vi "Calibration.vi"(4 "flush duration [s]":dbl, 6 "Exposure":sgl=50.0 format="%#_g ms", 7 "Desired Refresh Ratio":dbl=25.0 format="%#_g %", 8 "LINX Resource":T2={"IO"=enum."Remote", "Interface"=enum."TCP", "LINX Device Config"={"Interface"=enum."Serial", "COM Port"="COM13", "TCP Configuration"={"IP Address"="", "Port"=0}, "Device Family"=1, "Device ID"=1, "Device Name"="myRIO-1900", "TCP Ref"=refnum, "Channels"={"DI"=[0, 1, 2, 3, 4, 5, 6, 7, 8, 9, 10, 11, 12, 13, 14, 15, 16, 17, 18, 19, 20, 21, 22, 23, 24, 25, 26, 27, 28, 29, 30, 31, 32, 33, 34, 35, 36, 37, 38, 39, 40, 41, 42, 43, 44, 45, 46], "DO"=[0, 1, 2, 3, 4, 5, 6, 7, 8, 9, 10, 11, 12, 13, 14, 15, 16, 17, 18, 19, 20, 21, 22, 23, 24, 25, 26, 27, 28, 29, 30, 31, 32, 33, 34, 35, 36, 37, 38, 39, 40, 41, 42, 43, 44, 45, 46], "AI"=[0, 1, 2, 3, 4, 5, 6, 7, 8, 9, 10, 11], "AO"=[], "PWM"=[3, 5, 6, 9, 10], "QE"=[], "UART"=[0, 1], "I2C 2"=[0], "SPI"=[0], "CAN"=[], "Servo"=[], "AI Ref (V)"=0.0, "AI Resolution (Bits)"=0, "AO Ref (V)"=0.0, "AO Resolution (Bits)"=0}}}, 9 "SOLA ID":u32, 10 "TANGO ID":i32, 11 "IX 81 Port":refnum<visa-resource-name>="IX2-UCB") -> (0 "error IO":errorcluster, 2 "CalibFile":path, 3 "Number of pump steps\n for the desired refresh ratio":dbl)   [LabVIEW 2018]
doc: "This template is for the Queued Message Handler design pattern.\n\nThe Event Handling Loop generates messages based on user interface actions.\n\nThe Message Handling Loop processes messages generated by the Event Handling Loop, or by other messages. The messages are string values, so new messages can be added easily to the Message Cases case structure in the Message Handling Loop. Each message cluster can also provide an optional value for Message Data, which is a variant that can be converted to whatever message-specific data is required."
uses:
  <vilib>/MakerHub/LINX/Private/Type Defs/LINX Ref.ctl
  <vilib>/MakerHub/LINX/Private/Type Defs/Platform.ctl
  <vilib>/MakerHub/LINX/Private/Type Defs/Interface.ctl
  <vilib>/MakerHub/LINX/Private/Device/Type Defs/LINX Device Config.ctl
  <vilib>/MakerHub/LINX/Private/Device/Type Defs/TCP Config.ctl
  <vilib>/MakerHub/LINX/Private/Device/Type Defs/Channels.ctl
  C:/Users/johan/Downloads/LabVIEW software/LabVIEW software/IX-81 Software/lib/tiff/LVTiffWriter/BitMiracle.LibTiff.NET.dll
  lib/tiff/LVTiffWriter/BitMiracle.LibTiff.NET.dll
  <vilib>/MakerHub/LINX/Public/Peripherals/Digital/Digital Write N Chans.vi
  <vilib>/MakerHub/LINX/Private/Local IO/LinxDigitalWrite.vi
  <vilib>/MakerHub/LINX/Public/Utilities/Check Channel.vi
  <vilib>/MakerHub/LINX/Private/Utilties/Generate Error.vi
  lib/SOLA/LabVIEW 2015 Library (32bit)/LumencorDLL32/LumencorDLL32.lvlib
  lib/Olympus IX BX Series/Olympus IX BX Series.lvlib
  <vilib>/MakerHub/LINX/LMH-LINX.lvlib
  lib/ANDOR/Andor SDK/AndorSDK.lvlib
  <vilib>/vision/NI_Vision_Development_Module.lvlib
  lib/tiff/LVTiffWriter/LVTiffWriter.lvlib
  <vilib>/MakerHub/LINX/Private/Device/Device.lvlib
panel:
  out "function return":u32
  out "color":string
  in  "Messages":string
  out "TiffHandle":refnum<k24>
  in  "Image Name":string="TestIMG"
  out "Acq. Error Array":cluster{i32, string}[](array[cluster])
  in  "Single Image":bool
  out "Image":T1(plugin-control)
  in  "Colormap":u16(ring) items=["Grey", "Hot"]
  in  "Format":u16(ring)=6
  in  "Path":path
  in  "Save Image":bool
  in  "Exposure 2":sgl=50.0 format="%#_g ms"
  in  "Filter":u16(ring) items=["UV ", "CFP", "GFP", "YFP", "RFP", "BF (empty)"]
  out "exposure out":sgl
  out "accumulate out":sgl
  out "kinetic out":sgl
  out "Camera Temperature":sgl format="%.2f °C"
  in  "Calibrate at Startup":bool
  out "Y Limits":dbl[](array[numeric]) caption="Y Limits [µm]" format="%#_12f"
  out "X Limits":dbl[](array[numeric]) caption="X Limits [µm]" format="%#_10f"
  out "Lower Limit":dbl
  out "Upper Limit":dbl
  in  "Focus [um]":dbl format="%.3f"
  in  "Intensity [%]":dbl(slide) scale=0.0..100.0 scale format="%.1f"
  in  "Light Source":u16(ring) items=["BF - Lamp", "SOLA"]
  in  "Prism Position (1: Bi)":enum16{"Bi", "Side"}(ring)=enum."Side"
  in  "Objective":enum16{"x 4", "x 10", "x 20", "x 40", "x 100"}(ring)=enum."x 10"
  in  "Lamp Type (0: Transmitted)":enum16{"Transmitted", "Reflected"}(ring)
  in  "Enable Lamp":bool
  in  "Shutter":bool
  in  "Microscope Settings":i32(listbox)
  out "Slide":u8(slide) scale=0.0..100.0
  in  "Valve Actuation":i32(listbox)
  in  "Configuration File Path":path
  in  "stop":bool
  out "error out":errorcluster
  in  "Position List":i32[](listbox)
  out "Tango Success":bool
  in  "TANGO COM Port":refnum<visa-resource-name>="COM4"
  in  "SOLA COM Port":refnum<visa-resource-name>="COM5"
  in  "Valve Port (Arduino)":refnum<visa-resource-name>="COM7"
  # "Initialization"
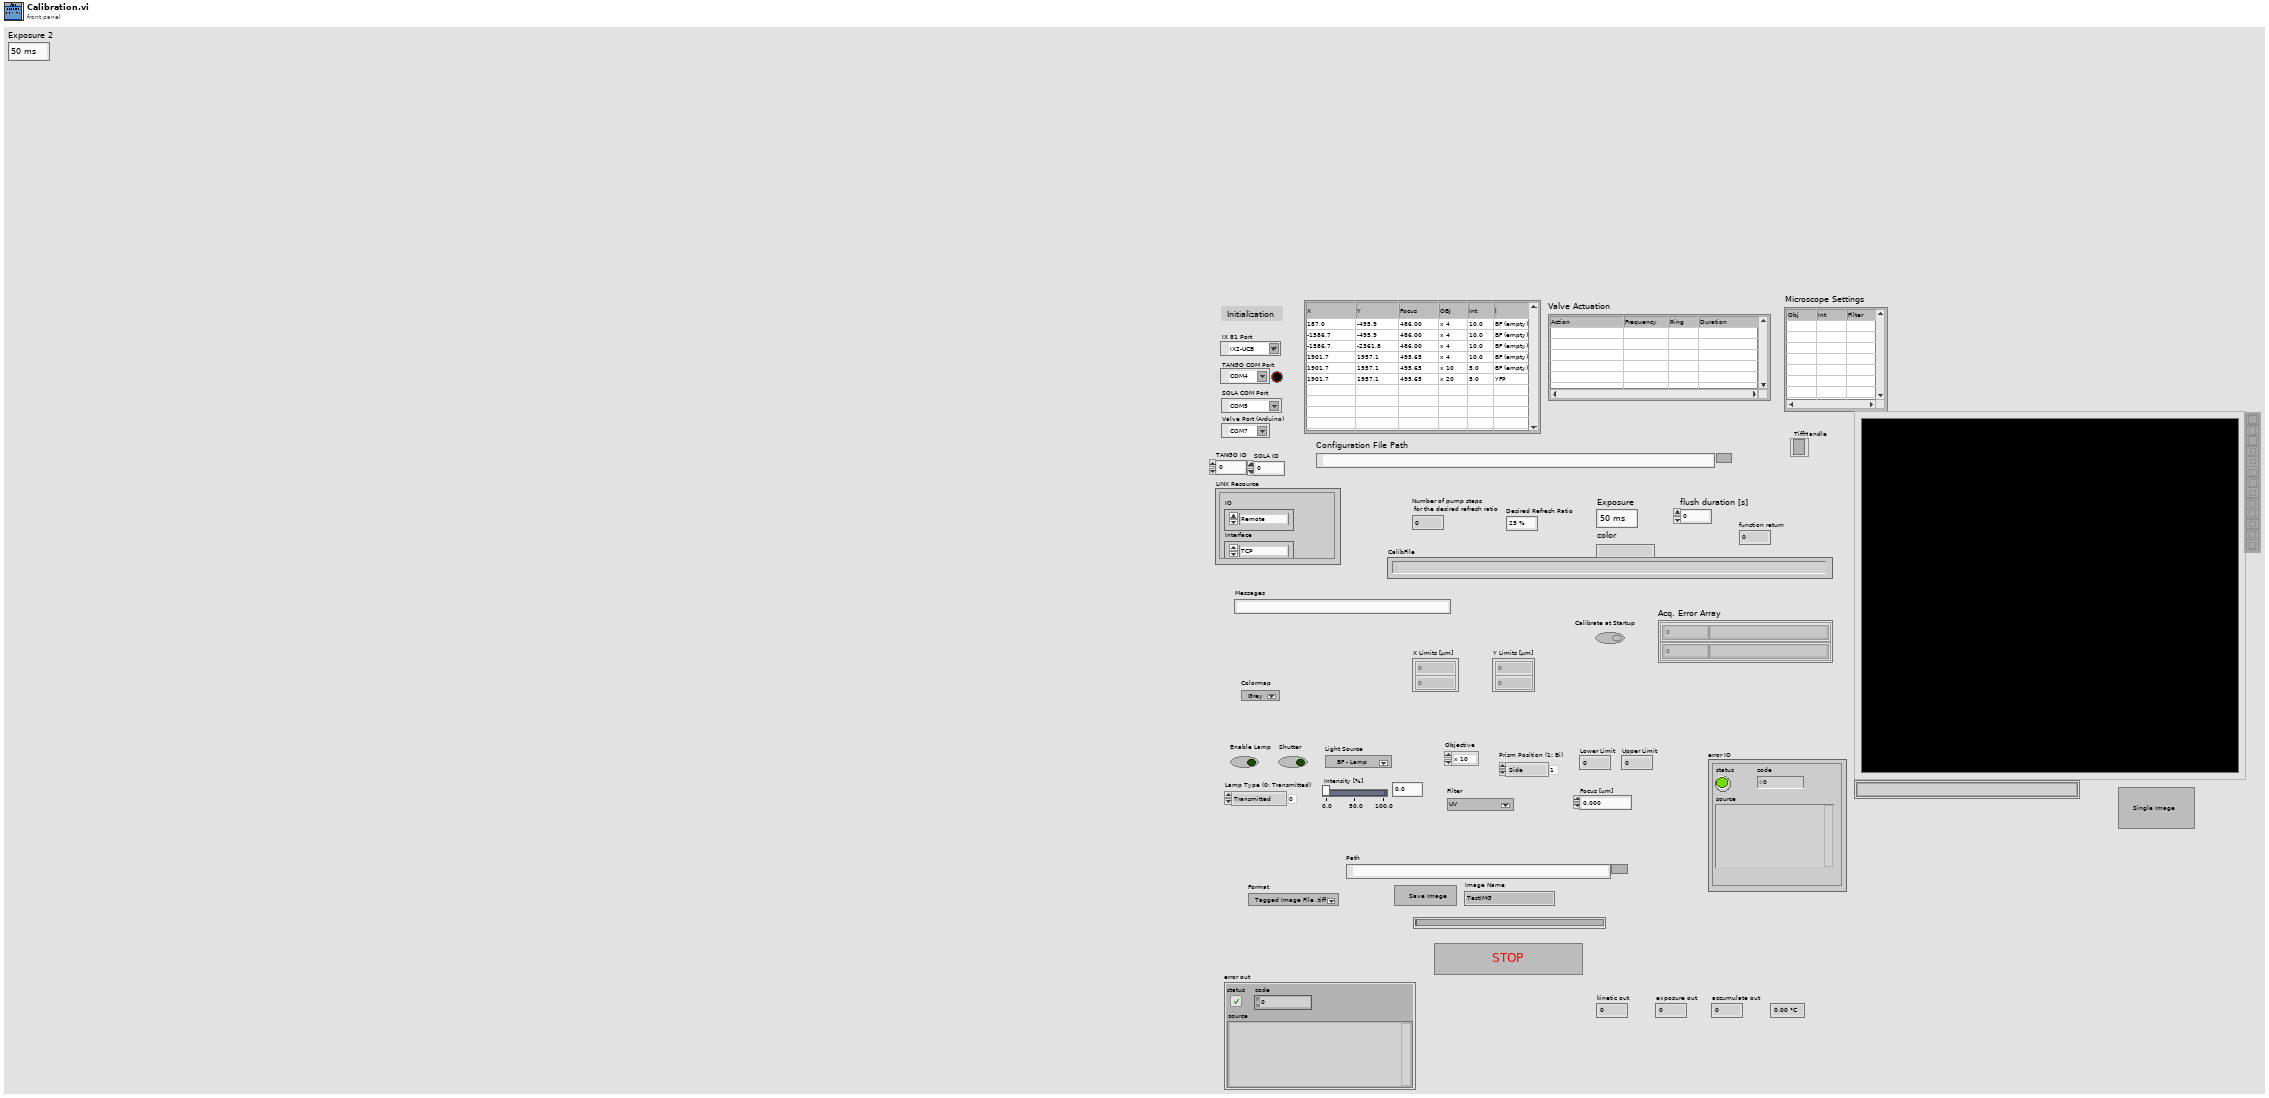
[diagram p1: front panel]
types:
  T1 = typedef "IMAQ Image.ctl" = refnum<image>
  T2 = typedef "LMH-LINX.lvlib/LINX Ref.ctl" = cluster{"IO":T3, "Interface":T4, "LINX Device Config":T5}
  T3 = typedef "LMH-LINX.lvlib/Platform.ctl" = enum16{"Remote", "Local"}
  T4 = typedef "LMH-LINX.lvlib/Interface.ctl" = enum16{"Serial", "TCP"}
  T5 = typedef "LMH-LINX.lvlib/Device.lvlib/LINX Device Config.ctl" = cluster{"Interface":T4, "COM Port":refnum<visa-resource-name>, "TCP Configuration":T6, "Device Family":u8, "Device ID":u8, "Device Name":string, "TCP Ref":refnum<k5>, "Channels":T7}
  T6 = typedef "LMH-LINX.lvlib/Device.lvlib/TCP Config.ctl" = cluster{"IP Address":string, "Port":u16}
  T7 = typedef "LMH-LINX.lvlib/Channels.ctl" = cluster{"DI":u8[], "DO":u8[], "AI":u8[], "AO":u8[], "PWM":u8[], "QE":u8[], "UART":u8[], "I2C 2":u8[], "SPI":u8[], "CAN":u8[], "Servo":u8[], "AI Ref (V)":dbl, "AI Resolution (Bits)":u8, "AO Ref (V)":dbl, "AO Resolution (Bits)":u8}
  T8 = enum16{"open", "replace", "create", "open or create", "replace or create", "replace or create with confirmation"}
  T9 = typedef "Image Type" = u32
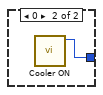
[diagram p2: hidden frame]
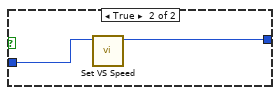
[diagram p3: hidden frame]
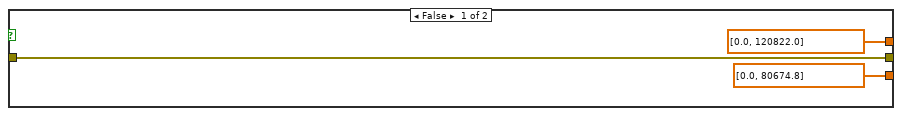
[diagram p4: hidden frame]
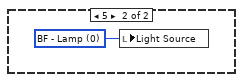
[diagram p5: hidden frame]
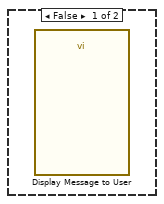
[diagram p7: hidden frame]
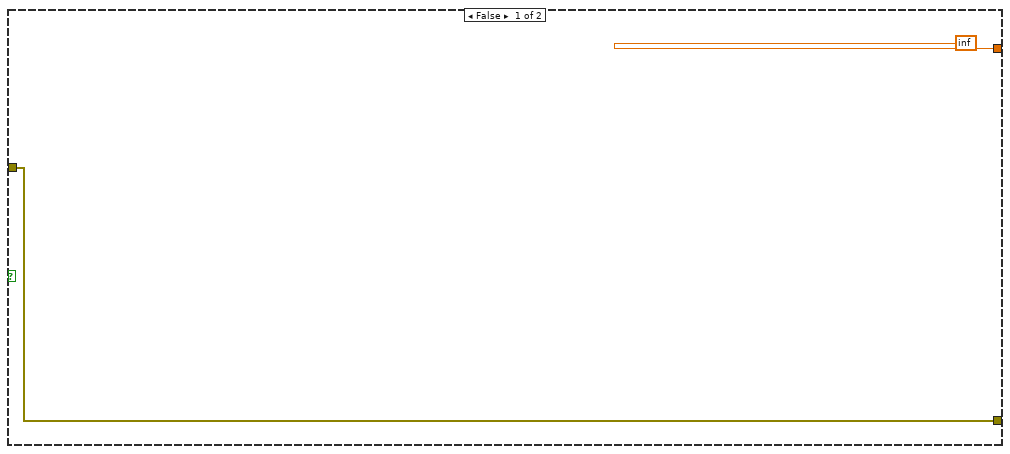
[diagram p11: hidden frame]
diagram:
  n1 = flat-sequence {
    tunnel: [errorcluster {"status"=FALSE, "code"=0, "source"=""} ("error IO")] -> w2
    tunnel: w2 -> [w5]
    tunnel: [w4] -> w1
    tunnel: w1 -> [_]
    frame #0 {
    }
    frame #1 {
      w70 = 0  # openingtime
      w68 = 0  # Auto Mode
      w67 = 1  # TTL High to open
      w69 = 0  # closingtime
      w66 = 0  # Internal Trigger
      w64 = 1  # Single Scan
      w65 = 4  # Image Read
      n2 = local read "IX 81 Port"() -> (w152:refnum<visa-resource-name>)
      n3 = call "Set Temperature.vi"("temperature"=-60) -> ()  [unwired: 10 in, 1 out]
      n4 = local write "Upper Limit"(3000000.0 ("default (0 I32)")) -> ()
      n5 = call "Set Active Objective.vi"("error in (no error)"=w5, "Objective Number (1)"=1, "Device Number (1)"=1, "VISA Resource Name"=w152) -> ("error out"=w103:errorcluster, "VISA Resource Name Out"=w104:refnum<visa-resource-name>)  [unwired: 6 in]
      n6 = local write "Lower Limit"(10.0 ("Upper Limit")) -> ()
      n7 = call "OlympusQuery.vi"("error in (no error)"=w103, "String"="SW OFF", "VISA Resource Name In"=w104) -> ("error out"=w107:errorcluster, "VISA Resource Name Out"=w108:refnum<visa-resource-name>)  [unwired: 6 in, 1 out]
      n8 = call "Is Cooler On.vi"() -> ("function return"=w53:u32, "iCoolerStatus out"=w54:i32)  [unwired: 10 in]
      n9 = call "OlympusQuery.vi"("error in (no error)"=w107, "String"="LMPSW OFF", "VISA Resource Name In"=w108) -> ("error out"=w102:errorcluster, "VISA Resource Name Out"=w149:refnum<visa-resource-name>)  [unwired: 6 in, 1 out]
      n10 = case shown="1, Default" w54 {
        tunnel: [u32 20002 ("function return") w161] -> w52
        frame 1, Default {
        }
        frame 0 {
          n11 = call "Cooler ON.vi"() -> ("function return"=w161:u32)  [unwired: 11 in]
        }
      }
      n12 = call "Get VS Speed.vi"() -> ("speed out"=w73:sgl, "function return"=w40:u32)  [unwired: 10 in]
      n13 = call "Get Fastest Recommended VS Speed.vi"() -> ("function return"=w39:u32, "speed out"=w72:sgl, "index out"=w75:i32)  [unwired: 9 in]
      n14 = Greater Or Equal?(x=w72, y=w73) -> (x >= y?=w74:bool)
      n15 = call "OlympusQuery.vi"("error in (no error)"=w102, "String"="LMP?", "VISA Resource Name In"=w149) -> ("error out"=w100:errorcluster, "Result"=w110:string, "VISA Resource Name Out"=w148:refnum<visa-resource-name>)  [unwired: 6 in]
      n16 = call "AndorCreaterErrorCluster.vi"() -> ("Array"=w38:cluster{i32, string}[])  [unwired: 11 in]
      n17 = case shown="False" w74 {
        tunnel: w75 -> [_ w164]
        tunnel: [u32 20002 ("function return") w163] -> w41
        frame False {
        }
        frame True {
          n18 = call "Set VS Speed.vi"("index"=w164) -> ("function return"=w163:u32)  [unwired: 10 in]
        }
      }
      n19 = call "AndorReturn2Error.vi"("Error List"=w38, "Camera return"=w53) -> ("error out"=w36:errorcluster, "Error List out"=w37:cluster{i32, string}[])  [unwired: 8 in]
      n20 = Decimal String To Number(string=w110, default (0L)=0.0 ("default (0 I32)")) -> (number=w112:dbl)  [unwired: 1 in, 1 out]
      n21 = call "AndorReturn2Error.vi"("error in (no error)"=w36, "Error List"=w37, "Camera return"=w52) -> ("error out"=w35:errorcluster, "Error List out"=w9:cluster{i32, string}[])  [unwired: 7 in]
      n22 = call "OlympusQuery.vi"("error in (no error)"=w100, "String"="SHUT1?", "VISA Resource Name In"=w148) -> ("error out"=w98:errorcluster, "Result"=w131:string, "VISA Resource Name Out"=w146:refnum<visa-resource-name>)  [unwired: 6 in]
      n23 = Divide(x=w112, y=1.2 ("x")) -> (x/y=w101:dbl)
      n24 = local write "Intensity [%]"(w101) -> ()
      n25 = call "AndorReturn2Error.vi"("error in (no error)"=w35, "Error List"=w9, "Camera return"=w39) -> ("error out"=w34:errorcluster, "Error List out"=w10:cluster{i32, string}[])  [unwired: 7 in]
      n26 = Equal?(x=w131, y="OUT") -> (x = y?=w99:bool)
      n27 = local write "Shutter"(w99) -> ()
      n28 = call "AndorReturn2Error.vi"("error in (no error)"=w34, "Error List"=w10, "Camera return"=w40) -> ("error out"=w33:errorcluster, "Error List out"=w11:cluster{i32, string}[])  [unwired: 7 in]
      n29 = call "OlympusQuery.vi"("error in (no error)"=w98, "String"="LMPSEL?", "VISA Resource Name In"=w146) -> ("error out"=w95:errorcluster, "Result"=w129:string, "VISA Resource Name Out"=w96:refnum<visa-resource-name>)  [unwired: 6 in]
      n30 = call "Get Temperature F.vi"() -> ("function return"=w42:u32, "temperature out"=w71:sgl)  [unwired: 10 in]
      n31 = local write "Camera Temperature"(w71) -> ()
      n32 = call "AndorReturn2Error.vi"("error in (no error)"=w33, "Error List"=w11, "Camera return"=w41) -> ("error out"=w32:errorcluster, "Error List out"=w12:cluster{i32, string}[])  [unwired: 7 in]
      n33 = Equal?(x=w129, y="DIA") -> (x = y?=w127:bool)
      n34 = call "AndorReturn2Error.vi"("error in (no error)"=w32, "Error List"=w12, "Camera return"=w42) -> ("error out"=w31:errorcluster, "Error List out"=w13:cluster{i32, string}[])  [unwired: 7 in]
      n35 = Not(x=w127) -> (.not. x?=w126:bool)
      n36 = call "OlympusQuery.vi"("error in (no error)"=w95, "String"="MU?", "VISA Resource Name In"=w96) -> ("error out"=w94:errorcluster, "Result"=w125:string, "VISA Resource Name Out"=w106:refnum<visa-resource-name>)  [unwired: 6 in]
      n37 = call "Set Read Mode.vi"("mode"=w65) -> ("function return"=w43:u32)  [unwired: 10 in]
      n38 = call "Set Shutter.vi"("openingtime"=w70, "closingtime"=w69, "mode"=w68, "typ"=w67) -> ("function return"=w44:u32)  [unwired: 7 in]
      n39 = Decimal String To Number(string=w125) -> (number=w124:i32)  [unwired: 2 in, 1 out]
      n40 = call "AndorReturn2Error.vi"("error in (no error)"=w31, "Error List"=w13, "Camera return"=w43) -> ("error out"=w30:errorcluster, "Error List out"=w14:cluster{i32, string}[])  [unwired: 7 in]
      n41 = Boolean To (0,1)(Boolean=w126) -> (0, 1=w97:i16)
      n42 = local write "Lamp Type (0: Transmitted)"(w97) -> ()
      n43 = call "OlympusQuery.vi"("error in (no error)"=w94, "String"="OB 2", "VISA Resource Name In"=w106) -> ("error out"=w93:errorcluster, "VISA Resource Name Out"=w141:refnum<visa-resource-name>)  [unwired: 6 in, 1 out]
      n44 = call "AndorReturn2Error.vi"("error in (no error)"=w30, "Error List"=w14, "Camera return"=w44) -> ("error out"=w29:errorcluster, "Error List out"=w15:cluster{i32, string}[])  [unwired: 7 in]
      n45 = call "Set Trigger Mode.vi"("mode"=w66) -> ("function return"=w45:u32)  [unwired: 10 in]
      n46 = Decrement(x=w124) -> (x-1=w105:i32)
      n47 = local write "Filter"(w105) -> ()
      n48 = call "AndorReturn2Error.vi"("error in (no error)"=w29, "Error List"=w15, "Camera return"=w45) -> ("error out"=w28:errorcluster, "Error List out"=w16:cluster{i32, string}[])  [unwired: 7 in]
      n49 = call "Set Acquisition Mode.vi"("mode"=w64) -> ("function return"=w46:u32)  [unwired: 10 in]
      n50 = call "AndorReturn2Error.vi"("error in (no error)"=w28, "Error List"=w16, "Camera return"=w46) -> ("error out"=w27:errorcluster, "Error List out"=w17:cluster{i32, string}[])  [unwired: 7 in]
      n51 = case shown="0, Default" w105 {
        frame 0, Default {
          w173 = u16 1 items=["BF - Lamp", "SOLA"] ("Light Source")
          n52 = local write "Light Source"(w173) -> ()
        }
        frame 5 {
          w174 = u16 0 items=["BF - Lamp", "SOLA"] ("Light Source")
          n53 = local write "Light Source"(w174) -> ()
        }
      }
      n54 = call "OlympusQuery.vi"("error in (no error)"=w93, "String"="PRISM?", "VISA Resource Name In"=w141) -> ("error out"=w92:errorcluster, "Result"=w123:string, "VISA Resource Name Out"=w140:refnum<visa-resource-name>)  [unwired: 6 in]
      n55 = Decimal String To Number(string=w123) -> (number=w122:i32)  [unwired: 2 in, 1 out]
      n56 = call "Set Frame Transfer Mode.vi"("mode"=1) -> ("function return"=w47:u32)  [unwired: 10 in]
      n57 = local read "Calibrate at Startup"() -> (w88:bool)
      n58 = call "OlympusQuery.vi"("error in (no error)"=w92, "Device Number\n(1: -Condensor\n     - Objective\n     - Lamp\n     - Shutter\n2: - Z-Motion\n   - Autofocus)"=2 ("Device Number\n(1: -Condensor\n     - Objective\n     - Lamp\n     - Shutter\n2: - Z-Motion\n   - Autofocus)"), "String"="FARLMT 10", "VISA Resource Name In"=w140) -> ("error out"=w137:errorcluster, "VISA Resource Name Out"=w138:refnum<visa-resource-name>)  [unwired: 5 in, 1 out]
      n59 = call "AndorReturn2Error.vi"("error in (no error)"=w27, "Error List"=w17, "Camera return"=w47) -> ("error out"=w26:errorcluster, "Error List out"=w18:cluster{i32, string}[])  [unwired: 7 in]
      n60 = Decrement(x=w122) -> (x-1=w91:i32)
      n61 = case shown="True" w88 {
        tunnel: [w165 w172] -> w77
        tunnel: w5 -> [w165 w168]
        tunnel: [dbl[] [0.0, 80674.8] ("Y Limits") w171] -> w86
        tunnel: [dbl[] [0.0, 120822.0] ("X Limits") w170] -> w87
        frame False {
        }
        frame True {
          n62 = local read "TANGO ID"() -> (w169:i32)
          n63 = call "TangoCalibrate.vi"("error in (no error)"=w168, "plLSID in"=w169) -> ("error out"=w172:errorcluster, "X Limits"=w170:dbl[], "Y Limits"=w171:dbl[])  [unwired: 7 in]
        }
      }
      n64 = local write "Prism Position (1: Bi)"(w91) -> ()
      n65 = call "Set Number Accumulations.vi"("number"=1) -> ("function return"=w48:u32)  [unwired: 10 in]
      n66 = local read "Exposure"() -> (w60:sgl)
      n67 = call "OlympusQuery.vi"("error in (no error)"=w137, "Device Number\n(1: -Condensor\n     - Objective\n     - Lamp\n     - Shutter\n2: - Z-Motion\n   - Autofocus)"=2 ("Device Number\n(1: -Condensor\n     - Objective\n     - Lamp\n     - Shutter\n2: - Z-Motion\n   - Autofocus)"), "String"="NEARLMT 3000000", "VISA Resource Name In"=w138) -> ("error out"=w134:errorcluster, "VISA Resource Name Out"=w135:refnum<visa-resource-name>)  [unwired: 5 in, 1 out]
      n68 = call "AndorReturn2Error.vi"("error in (no error)"=w26, "Error List"=w18, "Camera return"=w48) -> ("error out"=w25:errorcluster, "Error List out"=w19:cluster{i32, string}[])  [unwired: 7 in]
      n69 = Divide(x=w60, y=sgl 1000.0) -> (x/y=w59:sgl)
      n70 = call "Set Number Kinetics.vi"("number"=1) -> ("function return"=w49:u32)  [unwired: 10 in]
      n71 = call "AndorReturn2Error.vi"("error in (no error)"=w25, "Error List"=w19, "Camera return"=w49) -> ("error out"=w24:errorcluster, "Error List out"=w20:cluster{i32, string}[])  [unwired: 7 in]
      n72 = call "OlympusQuery.vi"("error in (no error)"=w134, "Device Number\n(1: -Condensor\n     - Objective\n     - Lamp\n     - Shutter\n2: - Z-Motion\n   - Autofocus)"=2 ("Device Number\n(1: -Condensor\n     - Objective\n     - Lamp\n     - Shutter\n2: - Z-Motion\n   - Autofocus)"), "String"="POS?", "VISA Resource Name In"=w135) -> ("error out"=w116:errorcluster, "Result"=w117:string, "VISA Resource Name Out"=w115:refnum<visa-resource-name>)  [unwired: 5 in]
      n73 = call "Set Exposure Time.vi"("time"=w59) -> ("function return"=w50:u32)  [unwired: 10 in]
      n74 = call "ArdnoValve2Linx.vi"("error in (no error)"=w5, "Valve (A1-C8),\n comma separated"="A1,A2,A3,A4,A5,A6,A7,A8,B1,B2,B3,B4,B5,B6,B7,B8,C1,C2,C3,C4,C5,C6,C7,C8" ("Valve (A1-C8),\n comma separated")) -> ("error out"=w83:errorcluster, "Closed State"=w82:bool[], "Linx Port"=w81:i32[])  [unwired: 7 in]
      n75 = call "Get Acquisition Timings.vi"() -> ("kinetic out"=w57:sgl, "accumulate out"=w55:sgl, "exposure out"=w56:sgl, "function return"=w51:u32)  [unwired: 8 in]
      n76 = call "lm Color Level.vi"("error in (no error)"=w5, "str_Level"="100", "str_Color"="WHITE") -> ("error out"=w156:errorcluster, "str_Color out"=w157:string)  [unwired: 6 in, 1 out]
      n77 = local write "exposure out"(w56) -> ()
      n78 = local write "accumulate out"(w55) -> ()
      n79 = local write "kinetic out"(w57) -> ()
      n80 = local read "LINX Resource"() -> (w85:T2)
      n81 = call "AndorReturn2Error.vi"("error in (no error)"=w24, "Error List"=w20, "Camera return"=w50) -> ("error out"=w23:errorcluster, "Error List out"=w21:cluster{i32, string}[])  [unwired: 7 in]
      n82 = Decimal String To Number(string=w117, default (0L)=0.0 ("default (0 I32)")) -> (number=w7:dbl)  [unwired: 1 in, 1 out]
      n83 = call "AndorReturn2Error.vi"("error in (no error)"=w23, "Error List"=w21, "Camera return"=w51) -> ("error out"=w22:errorcluster)  [unwired: 7 in, 1 out]
      n84 = call "lm Color Enable.vi"("error in (no error)"=w156, "str_State"="ON", "str_Color"=w157) -> ("error out"=w78:errorcluster)  [unwired: 6 in, 2 out]
      n85 = call "Configure Jog.vi"("VISA Resource Name"=w115, "Device Number (1)"=2, "Enabled (False)"=TRUE, "error in (no error)"=w116) -> ("error out"=w80:errorcluster)  [unwired: 10 in, 1 out]
      n86 = call-poly <vilib>:"Digital Write.vi"("Error In"=w83, "Values"=w82, "DO Channels"=w81, "LINX Resource"=w85) -> ("Error Out"=w79:errorcluster)  [unwired: 6 in, 1 out]
      n87 = Divide(x=w7, y=1000.0) -> (x/y=w6:dbl)
      n88 = Merge Errors(w80, w79, w78, w77, w22) -> (w4:errorcluster)
      n89 = local write "X Limits"(w87) -> ()
      n90 = local write "Y Limits"(w86) -> ()
      n91 = local write "Focus [um]"(w6) -> ()
    }
    frame #2 {
      n92 = Two Button Dialog(message="Do you want to calibrate the pumps now?") -> (T button?=w175:bool)  [unwired: 2 in]
      n93 = case shown="True" w175 {
        frame False {
        }
        frame True {
          n94 = flat-sequence {
            tunnel: [w415] -> w177
            tunnel: w177 -> [w423]
            frame #0 {
              n95 = Open/Create/Replace File(prompt="Specify the .tif file to save the images in.", operation (0:open)=T8."create", access (0:read/write)=enum16{"read/write", "read-only", "write-only"}."read/write") -> (refnum out=w181:refnum<file>, error out=w182:errorcluster)  [unwired: 3 in, 1 out]
              n96 = Close File(refnum=w181, error in=w182) -> (path=w180:path)  [unwired: 1 out]
              "CalibFile" <- w180
              n97 = call "tiffOpenForWrite.vi"("Path"=w180) -> ("TiffOut"=→"TiffHandle":refnum<k24>)  [unwired: 10 in]
            }
            frame #1 {
              w191 = u16 1 items=["BF - Lamp", "SOLA"] ("Light Source")
              n98 = local write "Light Source"(w191) -> ()
              n99 = property on="Filter" class="Ring (strict)"() -> ("Strings []"=w190:string[])  [unwired: 2 in, 2 out]
              n100 = call "Exposure Time check"() -> ("Color"=w185:string, "Exposure Time  [ms]"=w186:dbl)  [unwired: 16 in, 2 out]
              "color" <- w185
              n101 = Array Size(array=w190) -> (size(s)=w188:i32)
              n102 = for {
                N: w188 -> [_]
                tunnel: w190 -> [w202] mode=indexing
                tunnel: w185 -> [w201]
                tunnel: [w200] -> w187
                i -> [w200]
                stop <- w203 stop-if-true
                n103 = Equal?(x=w201, y=w202) -> (x = y?=w203:bool)
              }
              n104 = flat-sequence {
                tunnel: [w204] -> w192
                tunnel: w186 -> [w205]
                tunnel: w192 -> [w215]
                frame #0 {
                  n105 = while {
                    tunnel: w205 -> [w206]
                    tunnel: [w206] -> w204
                    stop <- w207 stop-if-true
                    n106 = call "Get Status.vi"() -> ("function return"=w213:u32, "status out"=w210:i32)  [unwired: 10 in]
                    n107 = Equal?(x=20073 ("status out"), y=w210) -> (x = y?=w209:bool)
                    n108 = Equal?(x=w213, y=20002 ("x")) -> (x = y?=w208:bool)
                    n109 = And(x=w209, y=w208) -> (x .and. y?=w207:bool)
                  }
                }
                frame #1 {
                  n110 = Divide(x=w215, y=sgl 1000.0) -> (x/y=w217:dbl)
                  n111 = call "Set Exposure Time.vi"("time"=w217) -> ("function return"=→"function return":u32)  [unwired: 10 in]
                }
              }
              n112 = local write "Exposure"(w186) -> ()
              n113 = Less?(x=w187, y=w188) -> (x < y?=w189:bool)
              n114 = case shown="True" w189 {
                tunnel: w187 -> [_ w196]
                frame False {
                  n115 = call "Display Message to User"() -> ()  [unwired: 10 in, 2 out]
                }
                frame True {
                  n116 = Increment(x=w196) -> (x+1=w195:i32)
                  n117 = Number To Decimal String(number=w195) -> (decimal integer string=w197:string)  [unwired: 1 in]
                  n118 = call <vilib>:"Space Constant.vi"() -> ("String"=w199:string)
                  n119 = local read "IX 81 Port"() -> (w193:refnum<visa-resource-name>)
                  n120 = Concatenate Strings("MU", w199, w197) -> (w194:string)
                  n121 = call "OlympusQuery.vi"("String"=w194, "VISA Resource Name In"=w193) -> ()  [unwired: 7 in, 3 out]
                }
              }
            }
            frame #2 {
              n122 = flat-sequence {
                tunnel: FALSE ("NewVal") -> [w226]
                tunnel: [w226] -> w221
                tunnel: [w230] -> w220
                tunnel: w221 -> [w230]
                tunnel: w218 -> [w231]
                tunnel: w220 -> [w232]
                frame #0 {
                  w224 = 1  # Single Scan
                  w225 = 4  # Image Read
                  n123 = call "Set Acquisition Mode.vi"("mode"=w224) -> ()  [unwired: 10 in, 1 out]
                  n124 = call "Set Read Mode.vi"("mode"=w225) -> ()  [unwired: 10 in, 1 out]
                  n125 = call "Set Number Accumulations.vi"("number"=1) -> ()  [unwired: 10 in, 1 out]
                  n126 = call "Set Number Kinetics.vi"("number"=1) -> ()  [unwired: 10 in, 1 out]
                }
                frame #1 {
                  n127 = local read "Exposure"() -> (w227:sgl)
                  n128 = Divide(x=w227, y=sgl 1000.0) -> (x/y=w229:sgl)
                  n129 = call "Set Exposure Time.vi"("time"=w229) -> ()  [unwired: 10 in, 1 out]
                }
                frame #2 {
                  n130 = case shown="True" w232 {
                    tunnel: w231 -> [_ w242]
                    frame False {
                    }
                    frame True {
                      n131 = flat-sequence {
                        tunnel: w242 -> [w243]
                        tunnel: [w245] -> w241
                        tunnel: [w244] -> w240
                        tunnel: w241 -> [w247]
                        tunnel: w240 -> [w248]
                        tunnel: [w248] -> w239
                        tunnel: [w247] -> w238
                        tunnel: w239 -> [w263]
                        tunnel: w238 -> [w262]
                        tunnel: [w263] -> w237
                        tunnel: [w262] -> w236
                        tunnel: [w258] -> w235
                        tunnel: [w259] -> w234
                        tunnel: w237 -> [w267]
                        tunnel: w236 -> [w265]
                        tunnel: w235 -> [w266]
                        tunnel: w234 -> [w269]
                        tunnel: [w269] -> w233
                        tunnel: w233 -> [w285]
                        frame #0 {
                          n132 = call "Start Acquisition.vi"() -> ("function return"=w246:u32)  [unwired: 11 in]
                          n133 = call "ConvertErrCodeToMessage.vi"("function return"=w246, "Array"=w243) -> ("Element Return"=w244:cluster{i32, string}, "Array out"=w245:cluster{i32, string}[])  [unwired: 8 in]
                        }
                        frame #1 {
                          n134 = while {
                            stop <- w249 stop-if-true
                            n135 = call "Get Status.vi"() -> ("function return"=w255:u32, "status out"=w252:i32)  [unwired: 10 in]
                            n136 = Equal?(x=20073 ("status out"), y=w252) -> (x = y?=w251:bool)
                            n137 = Equal?(x=w255, y=20002 ("x")) -> (x = y?=w250:bool)
                            n138 = And(x=w251, y=w250) -> (x .and. y?=w249:bool)
                          }
                        }
                        frame #2 {
                          n139 = Square(x=1024) -> (x^2=w256:i32)
                          n140 = Initialize Array(i16 0 ("element"), w256) -> (w257:i16[])
                          n141 = call "Get Most Recent Image16.vi"("size"=w256, "arr"=w257) -> ("function return"=w258:u32, "arr out"=w259:u16[])  [unwired: 7 in, 1 out]
                        }
                        frame #3 {
                          n142 = call "ConvertErrCodeToMessage.vi"("function return"=w266, "Array"=w265) -> ("Element Return"=w268:cluster{i32, string})  [unwired: 8 in, 1 out]
                          n143 = Build Array(w268, w267) -> (w264:cluster{i32, string}[])
                          n144 = local write "Acq. Error Array"(w264) -> ()
                        }
                        frame #4 {
                          w288 = u32 2 items=["Zero Order", "Bi-Linear", "Quadratic", "Cubic Spline"] ("Interpolation Type")
                          w287 = T9 7 items=["Grayscale (U8)", "Grayscale (I16)", "Grayscale (SGL)", "Complex (CSG)", "RGB (U32)", "HSL (U32)", "RGB (U64)", "Grayscale (U16)"] ("Image Type")
                          w286 = 1024 ("dimension size")
                          n145 = local read "Image Name"() -> (w284:string)
                          n146 = Reshape Array(w285, w286, w286) -> (w270:u16[][])
                          n147 = call "IMAQ Create"("Image Name"=w284, "Image Type"=w287) -> ("New Image"=w289:T1)  [unwired: 3 in, 1 out]
                          n148 = local read "TiffHandle"() -> (w275:refnum<k24>)
                          n149 = property on="Image" class="ImageControl"() -> ("Image Area Height"=w282:u32, "Image Area Width"=w283:u32)  [unwired: 2 in, 2 out]
                          n150 = call "IMAQ ArrayToImage"("Image Pixels (U16)"=w270, "Image"=w289) -> ("Image Out"=w273:T1)  [unwired: 8 in, 1 out]
                          n151 = call "IMAQ GetImageSize"("Image"=w273) -> ("Y Resolution"=w276:i32, "X Resolution"=w279:i32)  [unwired: 3 in, 1 out]
                          n152 = Divide(x=w276, y=w282) -> (x/y=w290:dbl)
                          n153 = Divide(x=w279, y=w283) -> (x/y=w291:dbl)
                          n154 = call "tiffWriteImaqToTiff.vi"("Multipage"=cluster{"Page":i32, "TotalPages":i32} {"Page"=10, "TotalPages"=0}, "ImaqIn"=w273, "TiffIn"=w275) -> ("ImaqOut"=w274:T1)  [unwired: 7 in, 1 out]
                          n155 = Max & Min(x=w290, y=w291) -> (max(x,y)=w281:dbl, min(x,y)=w277:dbl)
                          n156 = Divide(x=w279, y=w281) -> (x/y=w280:dbl)
                          n157 = Divide(x=w276, y=w277) -> (x/y=w278:dbl)
                          n158 = call "IMAQ Resample"("X Resolution"=w280, "Y Resolution"=w278, "Interpolation Type"=w288, "Image Src"=w274) -> ("Image Dst Out"=w271:T1)  [unwired: 6 in, 1 out]
                          n159 = local write "Image"(w271) -> ()
                        }
                      }
                    }
                  }
                }
              }
              n160 = call "AndorCreaterErrorCluster.vi"() -> ("Array"=w218:cluster{i32, string}[])  [unwired: 11 in]
            }
            frame #3 {
              n161 = Two Button Dialog(message="Start dilution. Please load the fluorophore now") -> (T button?=w293:bool)  [unwired: 2 in]
              n162 = case shown="True" w293 {
                frame False {
                }
                frame True {
                  n163 = flat-sequence {
                    tunnel: [w297] -> w296
                    tunnel: w296 -> [w303]
                    tunnel: [w303] -> w295
                    tunnel: w295 -> [w306]
                    tunnel: [w304] -> w294
                    frame #0 {
                      n164 = local read "LINX Resource"() -> (w301:T2)
                      n165 = call "ArdnoFlush.vi"("Open?"=FALSE, "Single / Multivalve?"=FALSE, "Channel"=u32 1, "LINX Resource"=w301) -> ("LINX Resource out"=w297:T2)  [unwired: 6 in, 1 out]
                    }
                    frame #1 {
                      n166 = Wait (ms)(milliseconds to wait="flush duration [s]") -> ()  [unwired: 1 out]
                    }
                    frame #2 {
                      (unwired) u32 1 ("Channel")
                      n167 = call "ArdnoFlush.vi"("Open?"=TRUE, "Single / Multivalve?"=FALSE, "LINX Resource"=w306) -> ("LINX Resource out"=w304:T2)  [unwired: 7 in, 1 out]
                    }
                  }
                  n168 = while {
                    tunnel: w294 -> [w315]
                    i -> [w312]
                    stop <- w309 continue-if-true
                    n169 = flat-sequence {
                      tunnel: w315 -> [w323]
                      tunnel: [w319] -> w314
                      tunnel: [w318] -> w313
                      tunnel: w314 -> [w328]
                      tunnel: w313 -> [w327]
                      tunnel: w312 -> [w329]
                      frame #0 {
                        n170 = call "ArdnoFeed.vi"("LINX Resource"=w323, "Single / Multivalve?"=FALSE, "Channel"=u32 1, "Feed Cycles"=15, "Frequency"=u32 8) -> ("LINX Resource out"=w319:T2, "error out"=w318:errorcluster)  [unwired: 9 in]
                      }
                      frame #1 {
                        n171 = call "ArdnoPump.vi"("LINX Resource"=w328, "Pump Cycles"=4, "Pump Frequency"=10, "error in (no error)"=w327, "Single/\nMultiring?"=FALSE ("Single/\nMultiring?")) -> ()  [unwired: 2 out]
                      }
                      frame #2 {
                        n172 = flat-sequence {
                          tunnel: TRUE ("NewVal") -> [w338]
                          tunnel: [w338] -> w333
                          tunnel: [w342] -> w332
                          tunnel: w333 -> [w342]
                          tunnel: w330 -> [w344]
                          tunnel: w332 -> [w345]
                          tunnel: w329 -> [w343]
                          frame #0 {
                            w336 = 1  # Single Scan
                            w337 = 4  # Image Read
                            n173 = call "Set Number Accumulations.vi"("number"=1) -> ()  [unwired: 10 in, 1 out]
                            n174 = call "Set Acquisition Mode.vi"("mode"=w336) -> ()  [unwired: 10 in, 1 out]
                            n175 = call "Set Read Mode.vi"("mode"=w337) -> ()  [unwired: 10 in, 1 out]
                            n176 = call "Set Number Kinetics.vi"("number"=1) -> ()  [unwired: 10 in, 1 out]
                          }
                          frame #1 {
                            n177 = local read "Exposure"() -> (w339:sgl)
                            n178 = Divide(x=w339, y=sgl 1000.0) -> (x/y=w341:sgl)
                            n179 = call "Set Exposure Time.vi"("time"=w341) -> ()  [unwired: 10 in, 1 out]
                          }
                          frame #2 {
                            n180 = case shown="True" w345 {
                              tunnel: w344 -> [_ w356]
                              tunnel: w343 -> [_ w346]
                              frame False {
                              }
                              frame True {
                                n181 = flat-sequence {
                                tunnel: w356 -> [w357]
                                tunnel: [w359] -> w355
                                tunnel: [w358] -> w354
                                tunnel: w355 -> [w361]
                                tunnel: w354 -> [w362]
                                tunnel: [w362] -> w353
                                tunnel: [w361] -> w352
                                tunnel: w353 -> [w377]
                                tunnel: w352 -> [w376]
                                tunnel: [w377] -> w351
                                tunnel: [w376] -> w350
                                tunnel: [w372] -> w349
                                tunnel: [w373] -> w348
                                tunnel: w351 -> [w381]
                                tunnel: w350 -> [w379]
                                tunnel: w349 -> [w380]
                                tunnel: w348 -> [w383]
                                tunnel: [w383] -> w347
                                tunnel: w347 -> [w406]
                                tunnel: w346 -> [w386]
                                frame #0 {
                                n182 = call "Start Acquisition.vi"() -> ("function return"=w360:u32)  [unwired: 11 in]
                                n183 = call "ConvertErrCodeToMessage.vi"("function return"=w360, "Array"=w357) -> ("Element Return"=w358:cluster{i32, string}, "Array out"=w359:cluster{i32, string}[])  [unwired: 8 in]
                                }
                                frame #1 {
                                n184 = while {
                                stop <- w363 stop-if-true
                                n185 = call "Get Status.vi"() -> ("function return"=w369:u32, "status out"=w366:i32)  [unwired: 10 in]
                                n186 = Equal?(x=20073 ("status out"), y=w366) -> (x = y?=w365:bool)
                                n187 = Equal?(x=w369, y=20002 ("x")) -> (x = y?=w364:bool)
                                n188 = And(x=w365, y=w364) -> (x .and. y?=w363:bool)
                                }
                                }
                                frame #2 {
                                n189 = Square(x=1024) -> (x^2=w370:i32)
                                n190 = Initialize Array(i16 0 ("element"), w370) -> (w371:i16[])
                                n191 = call "Get Most Recent Image16.vi"("size"=w370, "arr"=w371) -> ("function return"=w372:u32, "arr out"=w373:u16[])  [unwired: 7 in, 1 out]
                                }
                                frame #3 {
                                n192 = call "ConvertErrCodeToMessage.vi"("function return"=w380, "Array"=w379) -> ("Element Return"=w382:cluster{i32, string})  [unwired: 8 in, 1 out]
                                n193 = Build Array(w382, w381) -> (w378:cluster{i32, string}[])
                                n194 = local write "Acq. Error Array"(w378) -> ()
                                }
                                frame #4 {
                                w409 = u32 2 items=["Zero Order", "Bi-Linear", "Quadratic", "Cubic Spline"] ("Interpolation Type")
                                w408 = T9 7 items=["Grayscale (U8)", "Grayscale (I16)", "Grayscale (SGL)", "Complex (CSG)", "RGB (U32)", "HSL (U32)", "RGB (U64)", "Grayscale (U16)"] ("Image Type")
                                w407 = 1024 ("dimension size")
                                n195 = local read "Image Name"() -> (w405:string)
                                n196 = Reshape Array(w406, w407, w407) -> (w385:u16[][])
                                n197 = To Unsigned Word Integer(number=w385) -> (unsigned 16bit integer=w384:u16[][])
                                n198 = call "IMAQ Create"("Image Name"=w405, "Image Type"=w408) -> ("New Image"=w410:T1)  [unwired: 3 in, 1 out]
                                n199 = property on="Image" class="ImageControl"() -> ("Image Area Height"=w403:u32, "Image Area Width"=w404:u32)  [unwired: 2 in, 2 out]
                                n200 = call "IMAQ ArrayToImage"("Image Pixels (U16)"=w384, "Image"=w410) -> ("Image Out"=w390:T1)  [unwired: 8 in, 1 out]
                                n201 = call "IMAQ GetImageSize"("Image"=w390) -> ("Y Resolution"=w397:i32, "X Resolution"=w400:i32)  [unwired: 3 in, 1 out]
                                n202 = Add(x=1 ("y"), y=w386) -> (x+y=w391:i32)
                                n203 = Bundle By Name(cluster=cluster{"Page":i32, "TotalPages":i32} {"Page"=0, "TotalPages"=0} ("Multipage"), "TotalPages"=10, "Page"=w391) -> (w393:cluster{"Page":i32, "TotalPages":i32})
                                n204 = Divide(x=w397, y=w403) -> (x/y=w411:dbl)
                                n205 = Divide(x=w400, y=w404) -> (x/y=w412:dbl)
                                n206 = local read "TiffHandle"() -> (w395:refnum<k24>)
                                n207 = Max & Min(x=w411, y=w412) -> (max(x,y)=w402:dbl, min(x,y)=w398:dbl)
                                n208 = Divide(x=w400, y=w402) -> (x/y=w401:dbl)
                                n209 = Divide(x=w397, y=w398) -> (x/y=w399:dbl)
                                n210 = call "tiffWriteImaqToTiff.vi"("Multipage"=w393, "ImaqIn"=w390, "TiffIn"=w395) -> ("ImaqOut"=w389:T1, "TiffOut"=w396:refnum<k24>)  [unwired: 7 in]
                                n211 = local write "TiffHandle"(w396) -> ()
                                n212 = call "IMAQ Resample"("X Resolution"=w401, "Y Resolution"=w399, "Interpolation Type"=w409, "Image Src"=w389) -> ("Image Dst Out"=w388:T1)  [unwired: 6 in, 1 out]
                                n213 = local write "Image"(w388) -> ()
                                }
                                }
                              }
                            }
                          }
                        }
                        n214 = call "AndorCreaterErrorCluster.vi"() -> ("Array"=w330:cluster{i32, string}[])  [unwired: 11 in]
                      }
                    }
                    n215 = Not(x="stop") -> (.not. x?=w310:bool)
                    n216 = Less?(x=w312, y=10.0) -> (x < y?=w311:bool)
                    n217 = And(x=w311, y=w310) -> (x .and. y?=w309:bool)
                  }
                }
              }
            }
            frame #4 {
              n218 = local read "stop"() -> (w414:bool)
              n219 = case shown="True" w414 {
                tunnel: [w418 w421] -> w416
                tunnel: [inf w420] -> w415
                tunnel: errorcluster {"status"=FALSE, "code"=0, "source"=""} ("error constant") -> [w418 w419]
                frame False {
                }
                frame True {
                  n220 = script code="%% The aim of this script is to perform the calibration of the labview\n%  software with regards to the dilution volume as efficiently as possible\n%  requiring minimal input from the user. \n\n%% Set paths for Scripts and Functions\naddpath('C:\\Users\\e14user\\Documents\\LabVIEW software\\GitRepo\\Calibration')\naddpath C:\\Users\\johan\\Downloads\\LabVIEW software\\LabVIEW software\\IX-81 Software\\Calibration\naddpath C:\\Users\\Nikon\\Desktop\\Matlab_Calibration_Script\\20170421_CalibrationScript_V2\n\n\n%% Select the correct .Tiff file:\n[fileName,pathName,filterIndex] = uigetfile(\"*.tif\");\nimg = loadTiffFast([pathName,fileName]);\n\n%% Provide the Initial Concentration of Fluorophore\ncellConcentration = inputdlg({'Input Initial Fluorophore Concentration [µM]:'});\ninitialConcentration = str2double(cellConcentration{1,1});\n\n%% Set the intensity range with which to view all images during ROI selection\ndesiredIntensity = selectIntensity(img(:, :, 2));\nintensityRange = [0, desiredIntensity];\n\n%% ROI selection for all chambers\n% A figure will be shown of the first image taken by the microscope at each\n% of the locations of interest within the microfluidic device. Using the\n% cursor, select an ROI (Region of Interest) where the fluorescence\n% intensity will be determined. This area should fall within the boundaries\n% of the microfluidic flow channel. Draw the area by selecting the corners\n% of a polygon (left mouse click) and accept the polygon by\n% double-clicking within the borders of the polygon. \n[xCoordinates, yCoordinates] = regionOfInterestDetermination(img, intensityRange);\n\n%% Determine the intensities of the ROI within all images\nintensities = intensityDetermination(img, xCoordinates, yCoordinates);\n\n%% Plot the intensity curves and view the refresh ratio\n[final_Refresh_Ratio, refreshPerReactor] = plotIntensityCurves(intensities);\n% RR1 = refreshPerReactor(1,1)\n% RR2 = refreshPerReactor(2,1)\n% RR3 = refreshPerReactor(3,1)\n% RR4 = refreshPerReactor(4,1)\n% RR5 = refreshPerReactor(5,1)\n% RR6 = refreshPerReactor(6,1)\n% RR7 = refreshPerReactor(7,1)\n% RR8 = refreshPerReactor(8,1)\n\n%% This is the end of the script."("??"=w419) -> ("??"=w421:errorcluster, "refreshPerReactor"=w420:dbl)  [unwired: 1 out]
                }
              }
              "error IO" <- w416
            }
            frame #5 {
              n221 = Divide(x="Desired Refresh Ratio", y=w423) -> (x/y=w425:dbl)
              n222 = Multiply(x=15.0, y=w425) -> (x*y=w426:dbl)
              n223 = Round To Nearest(number=w426) -> (nearest integer value=→"Number of pump steps\n for the desired refresh ratio":dbl)
            }
          }
        }
      }
    }
  }
